vi "Get_Ch_data_from_file.vi"(0 "Filename":path, 9 "Channel names":string[](array[string]), 11 "Start of read offset (chars.: 0)":i32, 12 "Averaging Time(s)":dbl=5.0) -> (4 "exists?":bool, 6 "File Channels":string[](array[string]), 10 "Times":dbl[](array[numeric]) format="%.2f", 14 "stringArray":string[][](array[string]), 15 "Ch Data":dbl[][](array[numeric]) format="%.2f")   [LabVIEW 2022 SP3]
uses:
  <vilib>/Analysis/baseanly.llb/Mean (DBL).vi
  <vilib>/Analysis/NI_AALBase.lvlib
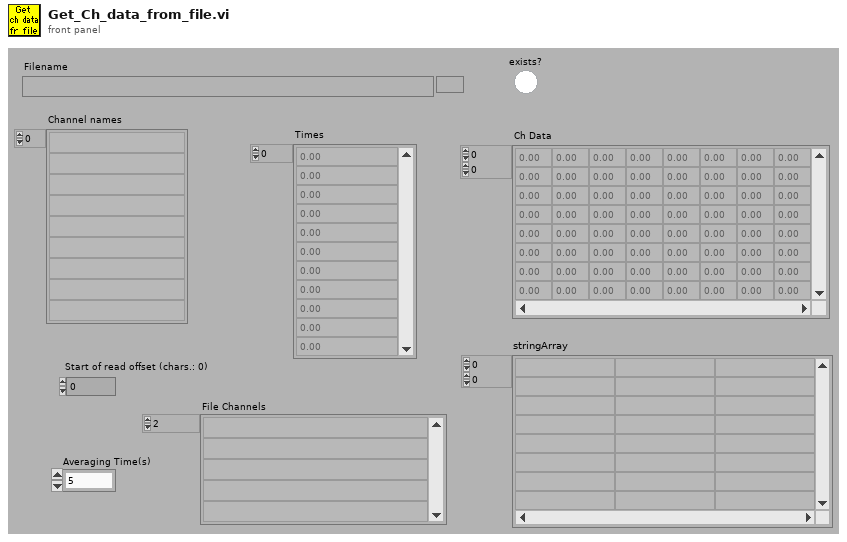
[diagram p1: front panel]
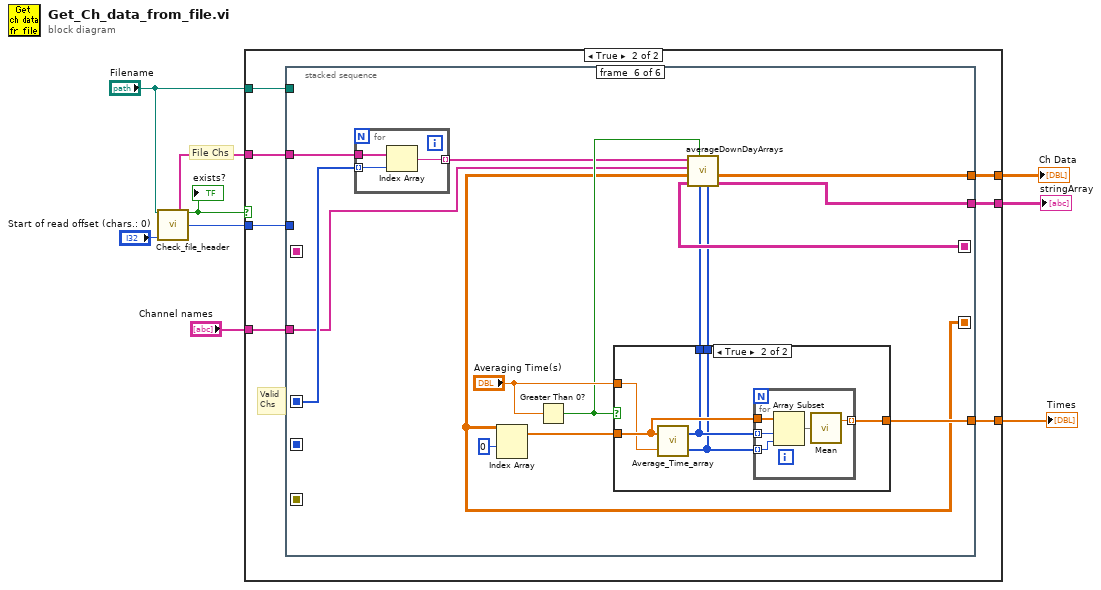
[diagram p0: block diagram]
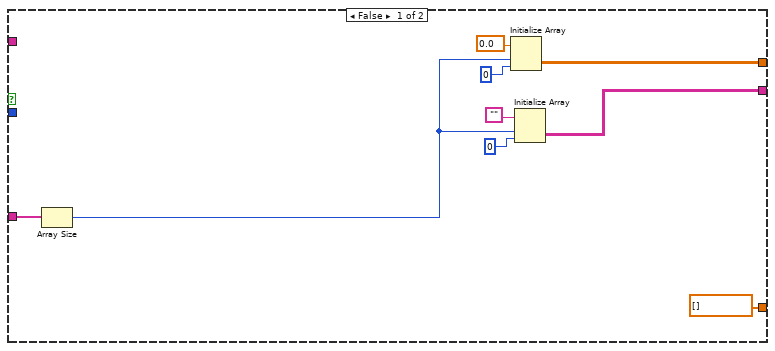
[diagram p2: hidden frame]
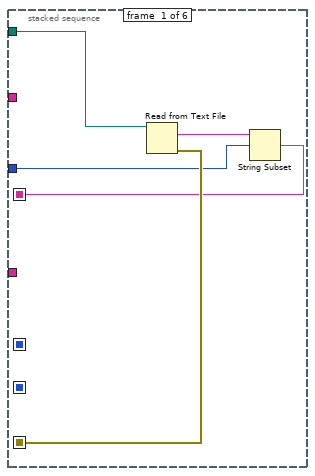
[diagram p3: hidden frame]
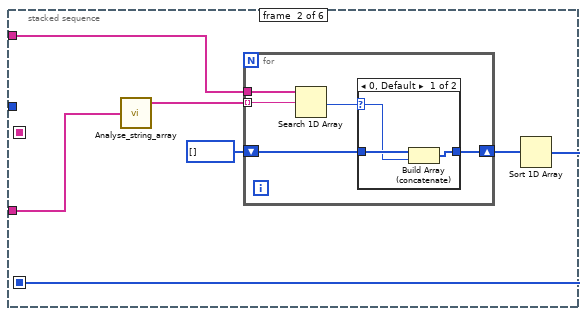
[diagram p4: hidden frame]
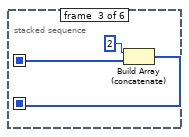
[diagram p6: hidden frame]
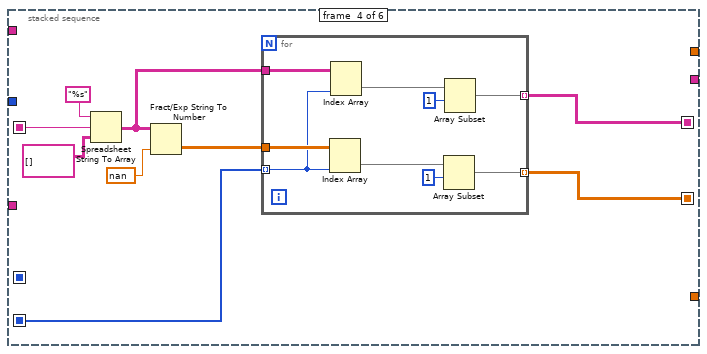
[diagram p7: hidden frame]
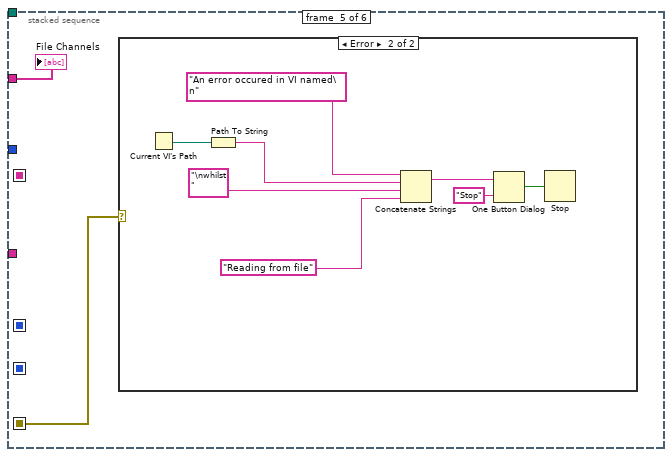
[diagram p8: hidden frame]
diagram:
  # "File Chs"
  n1 = call "Check_file_header.vi"("Filename"="Filename", "Start of read offset (chars.: 0)"="Start of read offset (chars.: 0)") -> ("File Channels"=w8:string[], "exists?"=w5:bool, "Start of data (bytes)"=w9:i64)  [unwired: 2 in, 9 out]
  "exists?" <- w5
  n2 = case shown="True" w5 {
    tunnel: w9 -> [_ w24]
    tunnel: w8 -> [_ w23]
    tunnel: "Filename" -> [_ w25]
    tunnel: [w14 w21] -> w4
    tunnel: [dbl[] [] w20] -> w3
    tunnel: "Channel names" -> [w15 w22]
    tunnel: [w10 w19] -> w1
    frame False {
      n3 = Array Size(array=w15) -> (size(s)=w11:i32)
      n4 = Initialize Array(0.0, w11, 0 ("Dimension Size")) -> (w14:dbl[][])
      n5 = Initialize Array("", w11, 0 ("Dimension Size")) -> (w10:string[][])
    }
    frame True {
      # "Valid\nChs"
      n6 = stacked-sequence {
        seq-local: [_ _ _ w54 _ _] -> [_ _ _ _ _ w81]
        seq-local: [_ _ w46 _ _ _] -> [_ _ _ w55 _ _]
        seq-local: [_ w33 _ _ _ _] -> [_ _ w47 _ _ w91]
        seq-local: [w26 _ _ _ _ _] -> [_ _ _ w56 _ _]
        seq-local: [w29 _ _ _ _ _] -> [_ _ _ _ w67 _]
        seq-local: [_ _ _ w49 _ _] -> [_ _ _ _ _ w82]
        tunnel: w25 -> [w30 _ _ _ _ _]
        tunnel: w24 -> [w27 _ _ _ _ _]
        tunnel: w23 -> [_ w36 _ _ w68 w90]
        tunnel: w22 -> [_ w32 _ _ _ w83]
        tunnel: [_ _ _ _ _ w80] -> w21
        tunnel: [_ _ _ _ _ w89] -> w20
        tunnel: [_ _ _ _ _ w79] -> w19
        frame #0 {
          n7 = Read from Text File(file (use dialog)=w30) -> (text=w28:string, error out=w29:errorcluster)  [unwired: 3 in, 2 out]
          n8 = String Subset(string=w28, offset (0)=w27) -> (substring=w26:string)  [unwired: 1 in]
        }
        frame #1 {
          n9 = call "Analyse_string_array.vi"("String array"=w32) -> ("Unique strings"=w31:string[])  [unwired: 2 out]
          n10 = for {
            tunnel: w36 -> [w41]
            tunnel: w31 -> [w40] mode=indexing
            shift-right: [w38] -> w34
            shift-left: i32[] [] -> [w39]
            n11 = Search 1D Array(1D array=w41, element=w40) -> (index of element=w37:i32)  [unwired: 1 out]
            n12 = case shown="0, Default" w37 {
              selector: w37 -> [w42 _]
              tunnel: w39 -> [w44 w45]
              tunnel: [w43 w45] -> w38
              frame 0, Default {
                n13 = Build Array (concatenate)(w44, w42) -> (w43:i32[])
              }
              frame -1 {
              }
            }
          }
          n14 = Sort 1D Array(array=w34) -> (sorted array=w33:i32[])
        }
        frame #2 {
          n15 = Build Array (concatenate)(2 ("t"), w47) -> (w46:i32[])
        }
        frame #3 {
          n16 = Spreadsheet String To Array(format string="%s", spreadsheet string=w56, array type (2D Dbl)=string[][] []) -> (array=w50:string[][])  [unwired: 1 in]
          n17 = Fract/Exp String To Number(string=w50, default (0 dbl)=nan ("default (0 DBL)")) -> (number=w51:dbl[][])  [unwired: 2 in, 1 out]
          n18 = for {
            tunnel: w55 -> [w59] mode=indexing
            tunnel: w51 -> [w66]
            tunnel: [w63] -> w54 mode=indexing
            tunnel: w50 -> [w60]
            tunnel: [w58] -> w49 mode=indexing
            n19 = Index Array(array=w66, index (col)=w59) -> (element=w65:dbl[])  [unwired: 1 in]
            n20 = Index Array(array=w60, index (col)=w59) -> (element=w61:string[])  [unwired: 1 in]
            n21 = Array Subset(array=w65, index=1) -> (w63:dbl[])  [unwired: 1 in]
            n22 = Array Subset(array=w61, index=1) -> (w58:string[])  [unwired: 1 in]
          }
        }
        frame #4 {
          n23 = case shown="Error" w67 {
            frame No Error {
            }
            frame Error {
              n24 = Current VI's Path() -> (path=w69:path)
              n25 = Path To String(path=w69) -> (string=w75:string)
              n26 = Concatenate Strings("An error occured in VI named\n", w75, "\nwhilst ", "Reading from file") -> (w73:string)
              n27 = One Button Dialog(message=w73, button name ("OK")="Stop") -> (true=w71:bool)
              n28 = Stop(stop? (T)=w71) -> ()
            }
          }
          "File Channels" <- w68
        }
        frame #5 {
          n29 = for {
            tunnel: w91 -> [w105] mode=indexing
            tunnel: w90 -> [w104]
            tunnel: [w103] -> w84 mode=indexing
            n30 = Index Array(array=w104, index=w105) -> (element=w103:string)
          }
          n31 = Index Array(array=w81, index (row)=0) -> (element=w86:dbl[])  [unwired: 1 in]
          n32 = Greater Than 0?(x="Averaging Time(s)") -> (x > 0?=w85:bool)
          n33 = case shown="True" w85 {
            tunnel: w86 -> [w92 w97]
            tunnel: [w92 w96] -> w89
            tunnel: [_ w94] -> w78
            tunnel: [_ w93] -> w77
            tunnel: "Averaging Time(s)" -> [_ w95]
            frame False {
            }
            frame True {
              n34 = call "Average_Time_array.vi"("Average TIme (seconds)"=w95, "Centre Time in Seconds"=w97) -> ("Length"=w93:i32[], "Start"=w94:i32[])
              n35 = for {
                tunnel: w97 -> [w102]
                tunnel: w94 -> [w101] mode=indexing
                tunnel: w93 -> [w100] mode=indexing
                tunnel: [w98] -> w96 mode=indexing
                n36 = Array Subset(array=w102, index=w101, length=w100) -> (w99:dbl[])
                n37 = call-poly <vilib>:"Mean.vi"("X"=w99) -> ("mean"=w98:dbl)  [unwired: 1 out]
              }
            }
          }
          n38 = call "averageDownDayArrays.vi"("Length"=w77, "Start"=w78, "averaging?"=w85, "textIn"=w82, "numericsIn"=w81, "requestedChannels"=w83, "goodChannels"=w84) -> ("textSummary"=w79:string[][], "numericAverages"=w80:dbl[][])  [unwired: 3 in]
        }
      }
    }
  }
  "Ch Data" <- w4
  "Times" <- w3
  "stringArray" <- w1
